vi "AC Test Host1.vi"() -> ()   [LabVIEW 2012]
uses:
  <vilib>/FPGAPlugInAG/PCI-7831R/niLvFpga_Open_PCI-7831R.vi
  <vilib>/rvi/interface/common/dynamic/niFpgaDynamicAddResources.vi
  <vilib>/Utility/error.llb/Error Cluster From Error Code.vi
  <vilib>/rvi/errors/niLvFpgaAdjustHostInterfaceError.vi
  <vilib>/FPGAPlugInAG/Dynamic/niLvFpga_Abort_Dynamic.vi
  <vilib>/FPGAPlugInAG/Dynamic/niLvFpga_Close_Dynamic.vi
  <vilib>/rvi/interface/nirviOpenFPGA/nirviOpenFPGA.xnode
  FPGA Bitfiles/Apporach-Retract_FPGATarget_InputOutputACSig_TqIhJi+rfhQ.lvbitx
  Input Output AC Signal Test1.vi
  <vilib>/rvi/interface/nirviReadWriteControl/nirviReadWriteControl.xnode
  <vilib>/rvi/interface/nirviMethod/nirviMethod.xnode
  <vilib>/rvi/interface/nirviCloseFPGA/nirviCloseFPGA.xnode
  NiFpgaLv.dll
  <vilib>/rvi/interface/Simulation/niFpgaSimulationCallBeginRW.vi
panel:
  out "Sine Output":sgl(graph)
  out "Sine Generator":dbl
  in  "Voltage":dbl
  in  "Frequency":dbl
  in  "Phase":dbl
  out "Sine Input":dbl(graph)
  out "Raw Sine Value":dbl
  in  "Stop":bool
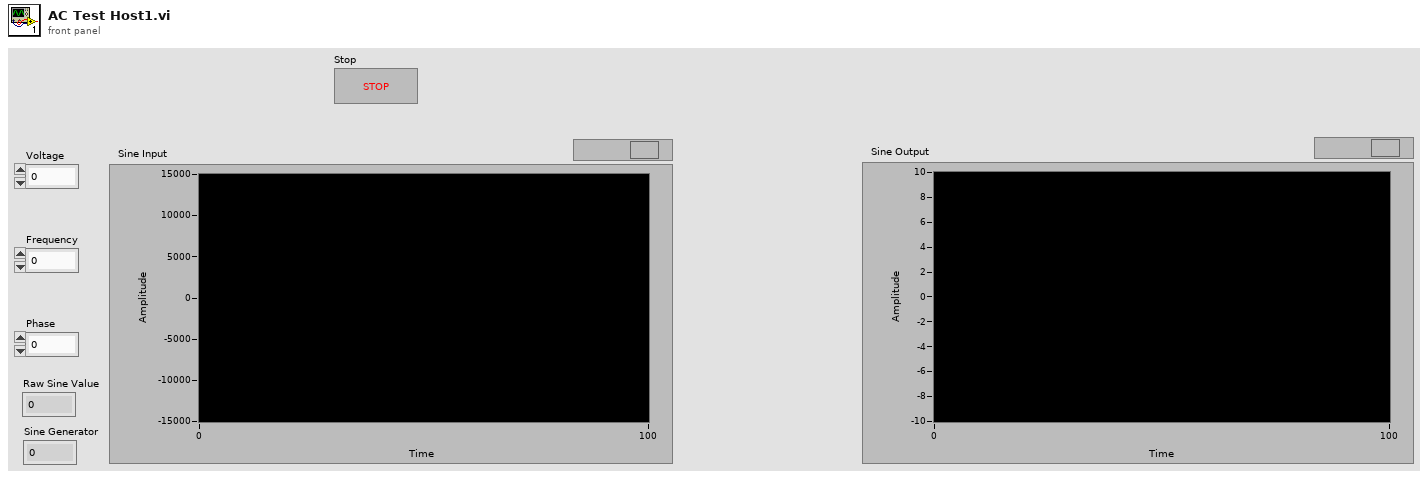
[diagram p1: front panel]
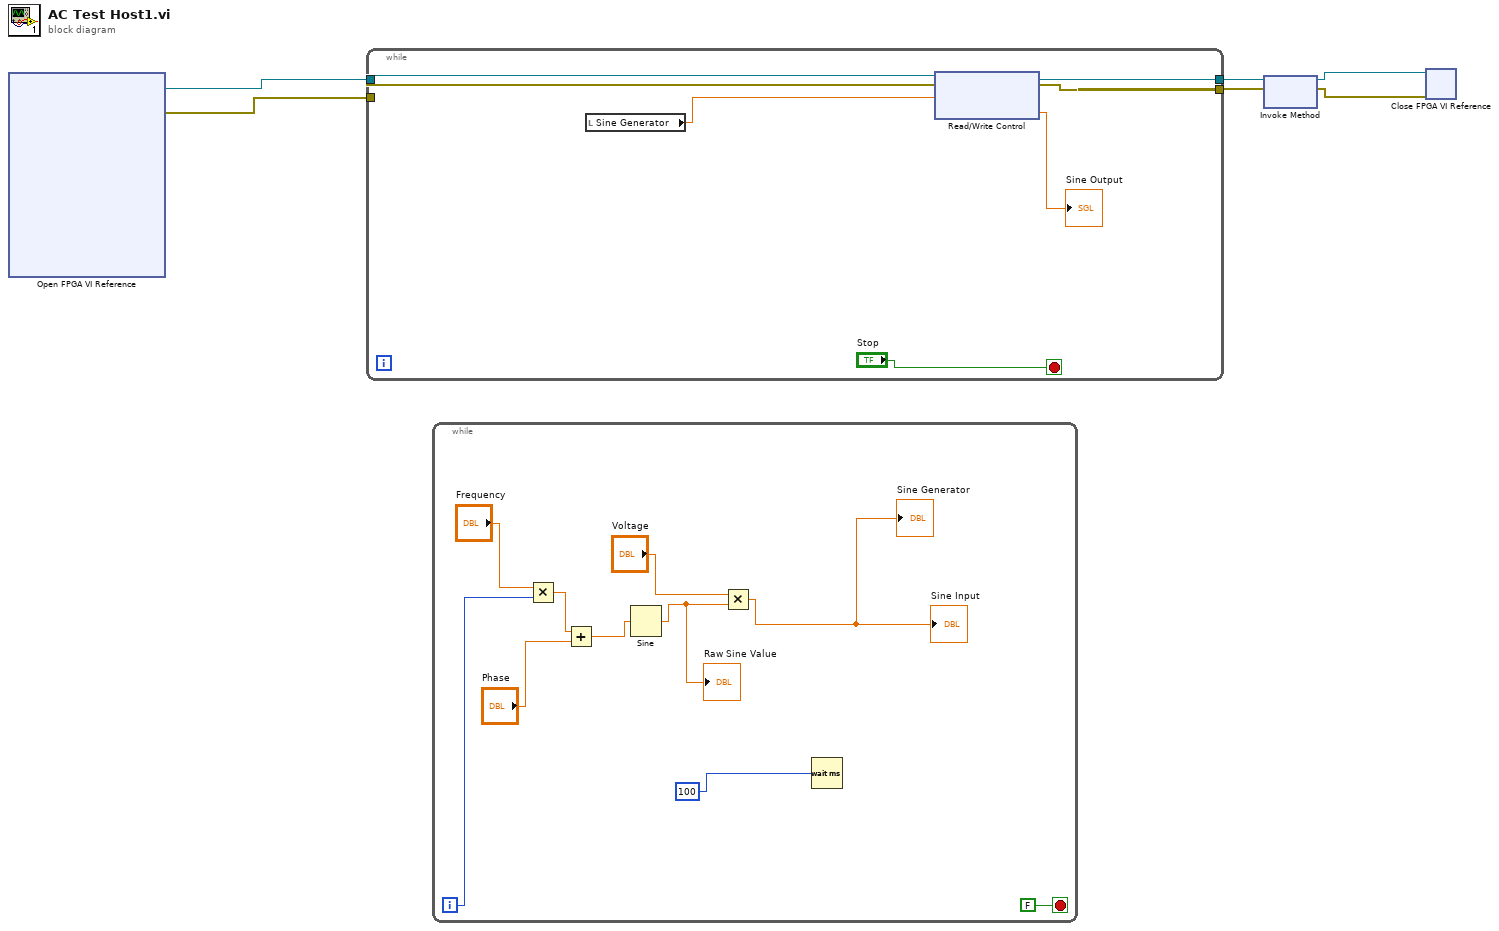
[diagram p0: block diagram]
diagram:
  n1 = xnode "Open FPGA VI Reference"() -> ("FPGA VI Reference Out"=w6:refnum<k20>, "error out"=w5:errorcluster)  [unwired: 2 in]
  n2 = while {
    tunnel: w6 -> [w13]
    tunnel: w5 -> [w12]
    tunnel: [w11] -> w4
    tunnel: [w10] -> w3
    stop <- "Stop" stop-if-true
    n3 = local read "Sine Generator"() -> (w8:dbl)
    n4 = xnode "Read/Write Control"("FPGA VI Reference In"=w13, "error in"=w12, "Sine Generator 2"=w8) -> ("FPGA VI Reference Out"=w11:refnum<k20>, "error out"=w10:errorcluster, "Output Signal 2"=→"Sine Output":sgl)
  }
  n5 = while {
    i -> [w17]
    stop <- FALSE stop-if-true
    n6 = Multiply(x="Frequency", y=w17) -> (x*y=w19:dbl)
    n7 = Add(x=w19, y="Phase") -> (x+y=w22:dbl)
    n8 = Sine(x=w22) -> (sin(x)=w15:dbl)
    "Raw Sine Value" <- w15
    n9 = Multiply(x="Voltage", y=w15) -> (x*y=→"Sine Input" →"Sine Generator":dbl)
    n10 = Wait (ms)(milliseconds to wait=100) -> ()  [unwired: 1 out]
  }
  n11 = xnode "Invoke Method"("FPGA VI Reference In"=w4, "error in"=w3) -> ("FPGA VI Reference Out"=w2:refnum<k20>, "error out"=w1:errorcluster)
  n12 = xnode "Close FPGA VI Reference"("FPGA VI Reference In"=w2, "error in"=w1) -> ()  [unwired: 1 out]
